vi "leds.vi"() -> ()   [LabVIEW 2020]
panel:
  in  "Latch Until Released":bool
  out "led 6":bool
  in  "Latch When Released":bool
  out "led 5":bool
  in  "Latch When Pressed":bool
  out "led 4":bool
  in  "Switch Until Released":bool
  out "led 3":bool
  in  "Switch when Released":bool
  out "led 2":bool
  in  "Switch when pressed":bool
  out "led 1":bool
  # "Modos de accion mecanica de los botones."
  # "1. En este modo el led enciende cuando se acciona el boton"
  # "2. En este modo el led enciende al soltar le boton."
  # "3. En este modo el estado del led cambia al ser soltado el boton"
  # "4. En este modo el estado del led cambia por un pequeño momento despues de precionar el boton."
  # "5. En este modo el led cambia su estado por un pequeño momento despues de liberar el boton."
  # "6. En este modo el led cambia por un momento hasta que se deja de precionar el boton."
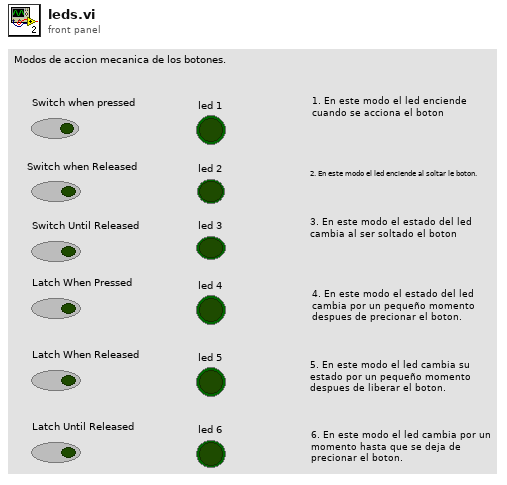
[diagram p1: front panel]
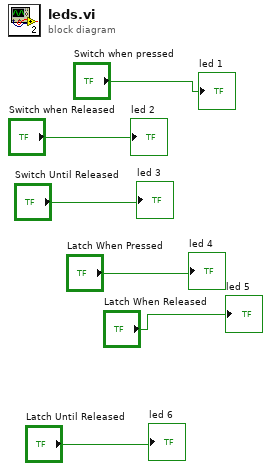
[diagram p0: block diagram]
diagram:
  "led 1" <- "Switch when pressed"
  "led 2" <- "Switch when Released"
  "led 3" <- "Switch Until Released"
  "led 4" <- "Latch When Pressed"
  "led 5" <- "Latch When Released"
  "led 6" <- "Latch Until Released"
